vi "add_int16.vi"   [LabVIEW 2014]
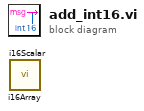
[diagram p0: block diagram]
diagram:
  n1 = call <userlib>:"i16Array.vi"() -> ()  [unwired: 5 in, 1 out]
  n2 = call <userlib>:"i16Scalar.vi"() -> ()  [unwired: 5 in, 1 out]
